vi "testMsgDetailsToJSON.vi"(8 "error in (no error)":errorcluster) -> (0 "error out":errorcluster)   [LabVIEW 2018]
doc: "Test the msgDetailsToJSON.vi."
uses:
  src/TcpServer/TcpServer.lvclass
  src/TcpServer/typedef/msgTypeDef.ctl
  src/TcpServer/typedef/msgTypeEnum.ctl
  <vilib>/addons/_JKI Toolkits/Caraya/classes/Assert/Assert Equal Value_Variant.vi
  <vilib>/addons/_JKI Toolkits/Caraya/classes/Assert/Assert Equal Value and Type_Variant.vi
  <vilib>/addons/_JKI Toolkits/Caraya/classes/Test/Test.lvclass
  <vilib>/addons/_JKI Toolkits/Caraya/classes/Assert/Assert.lvclass
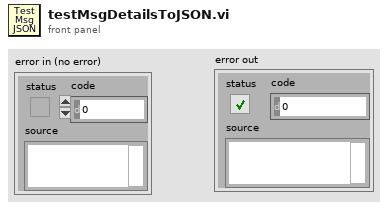
[diagram p1: front panel]
types:
  T1 = typedef "TcpServer.lvclass/msgTypeEnum.ctl" = enum16{"event", "telemetry"}
  T2 = typedef "TcpServer.lvclass/msgTypeDef.ctl" = cluster{"msgName":string, "msgDetails":string}
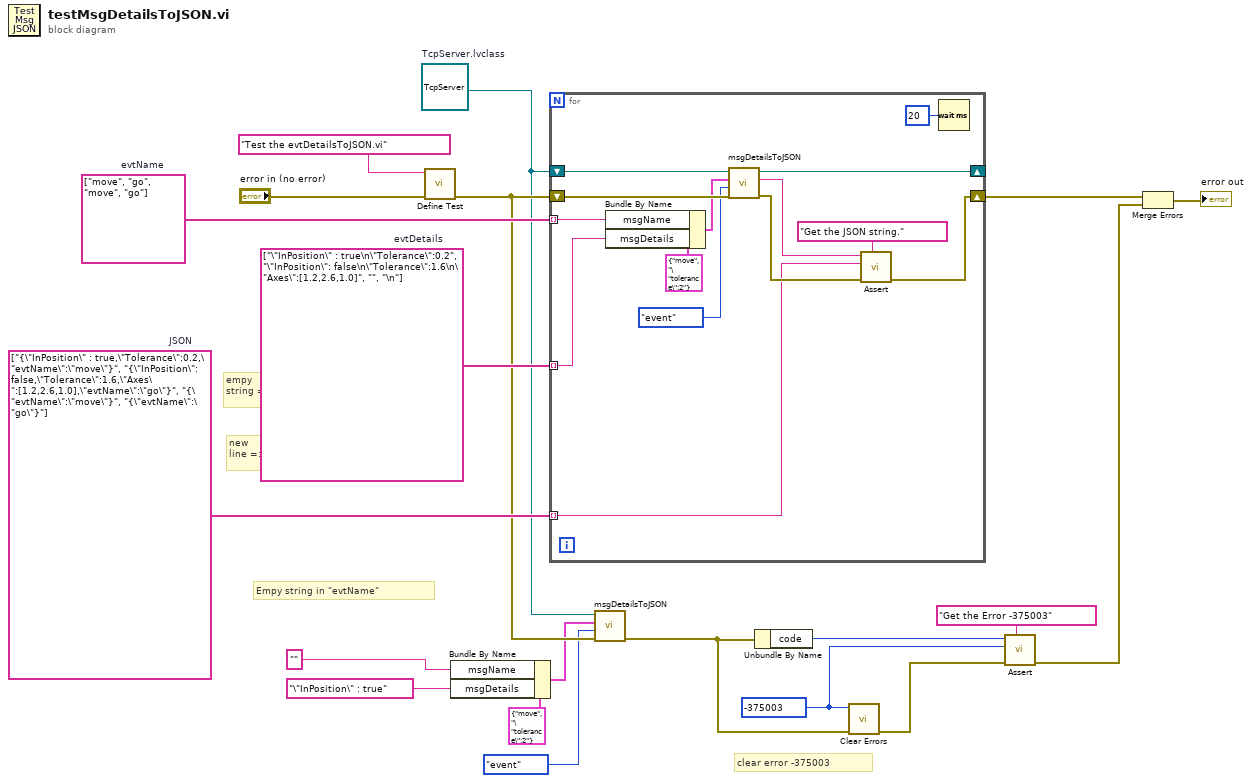
[diagram p0: block diagram]
diagram:
  w11 = -375003 ("code")
  w16 = string[] ["{\"InPosition\" : true,\"Tolerance\":0.2,\"evtName\":\"move\"}", "{\"InPosition\": false,\"Tolerance\":1.6,\"Axes\":[1.2,2.6,1.0],\"evtName\":\"go\"}", "{\"evtName\":\"move\"}", "{\"evtName\":\"go\"}"]  # JSON
  w17 = string[] ["\"InPosition\" : true\n\"Tolerance\":0.2", "\"InPosition\": false\n\"Tolerance\":1.6\n\"Axes\":[1.2,2.6,1.0]", "", "\n"]  # evtDetails
  w18 = string[] ["move", "go", "move", "go"]  # evtName
  w6 = refnum<class "TcpServer.lvclass"> refnum  # TcpServer.lvclass
  # "new \nline =>"
  # "empy \nstring =>"
  # "clear error -375003"
  # "Empy string in \"evtName\""
  n1 = call <vilib>:"Define Test.vi"("error in (no error)"="error in (no error)", "Label (VI Title)"="Test the evtDetailsToJSON.vi") -> ("error out"=w10:errorcluster)  [unwired: 9 in]
  n2 = Bundle By Name(cluster=T2 {"msgName"="move", "msgDetails"="\"tolerance\":2"} ("msgTypeDef"), "msgName"="" ("String"), "msgDetails"="\"InPosition\" : true" ("String")) -> (w4:T2)
  n3 = for {
    tunnel: w18 -> [w24] mode=indexing
    tunnel: w17 -> [w23] mode=indexing
    tunnel: w16 -> [w26] mode=indexing
    shift-right: [w27] -> w9
    shift-left: w10 -> [w33]
    shift-right: [w29] -> _
    shift-left: w6 -> [w34]
    n4 = Bundle By Name(cluster=T2 {"msgName"="move", "msgDetails"="\"tolerance\":2"} ("msgTypeDef"), "msgName"=w24, "msgDetails"=w23) -> (w22:T2)
    n5 = call "msgDetailsToJSON.vi"("error in (no error)"=w33, "msgTypeEnum"=msgTypeEnum."event", "msgTypeDef"=w22, "TcpServer.lvclass"=w34) -> ("error out"=w28:errorcluster, "JSON string"=w30:string, "TcpServer.lvclass"=w29:refnum<class "TcpServer.lvclass">)  [unwired: 5 in]
    n6 = call-poly <vilib>:"Assert.vi"("Label"="Get the JSON string.", "error in (no error)"=w28, "Y"=w26, "X"=w30) -> ("error out"=w27:errorcluster)  [unwired: 7 in]
    n7 = Wait (ms)(milliseconds to wait=u32 20) -> ()  [unwired: 1 out]
  }
  n8 = call "msgDetailsToJSON.vi"("error in (no error)"=w10, "msgTypeEnum"=msgTypeEnum."event", "msgTypeDef"=w4, "TcpServer.lvclass"=w6) -> ("error out"=w13:errorcluster)  [unwired: 5 in, 2 out]
  n9 = Unbundle By Name(w13) -> ("code"=w12:i32)
  n10 = call <vilib>:"Clear Errors.vi"("error in (no error)"=w13, "specific error code to clear (0: all)"=w11) -> ("error out"=w14:errorcluster)  [unwired: 4 in, 1 out]
  n11 = call-poly <vilib>:"Assert.vi"("Label"="Get the Error -375003", "error in (no error)"=w14, "Y"=w11, "X"=w12) -> ("error out"=w8:errorcluster)  [unwired: 7 in]
  n12 = Merge Errors(w9, w8) -> (→"error out":errorcluster)
